vi "AIT 1553 Initialization VI.vi"(8 "error in (no error)":errorcluster, 10 "Custom XML":string, 11 "Device Item Ref in":T1 format="%.0x") -> (0 "error out":errorcluster, 3 "Device Item Ref out":T1 format="%.0x")   [LabVIEW 2011, in "AIT 1553 Custom Device.lvlib"]
uses:
  AIT 1553 Custom Device.lvlib
  <vilib>/NI Veristand/Custom Device API/Custom Device Item Ref.ctl
  Controls and Global/Global.vi
  <vilib>/NI Veristand/Custom Device API/Custom Device API.lvlib
  <vilib>/NI Veristand/Custom Device Tools/Custom Device Utility Library/Custom Device Utility Library.lvlib
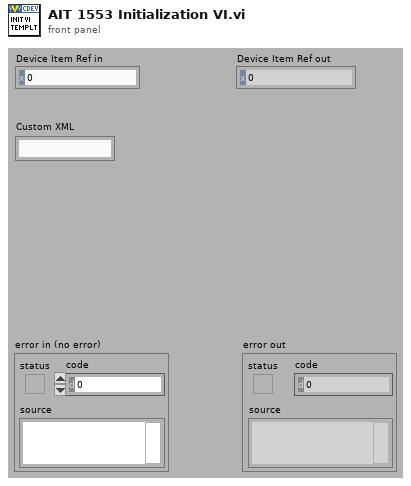
[diagram p1: front panel]
types:
  T1 = typedef "Custom Device API.lvlib/Custom Device Item Ref.ctl" = u64
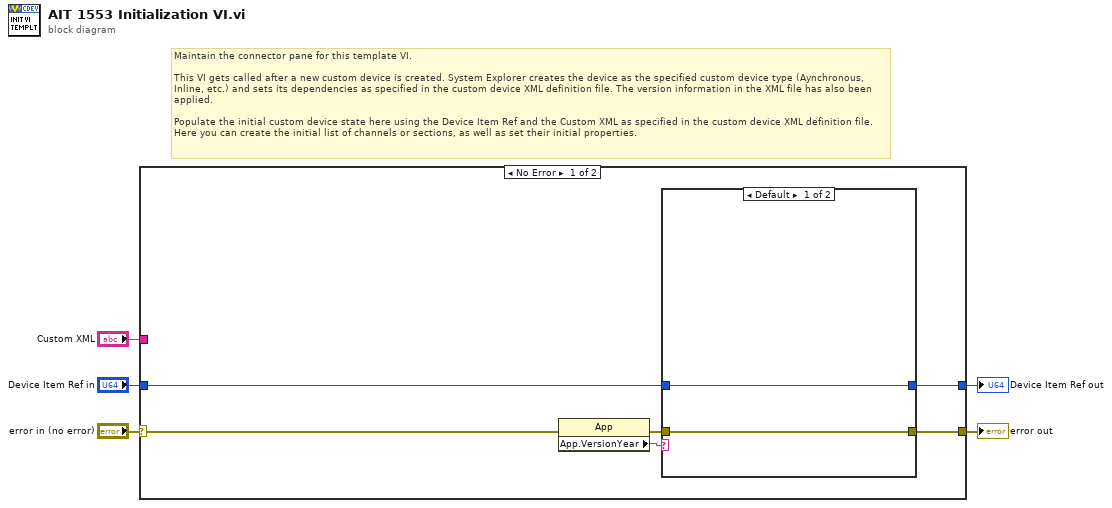
[diagram p0: block diagram]
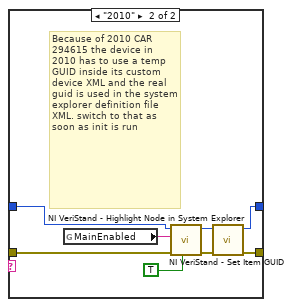
[diagram p2: hidden frame]
diagram:
  # "Maintain the connector pane for this template VI.\n\nThis VI gets called after a new custom device is created. System Explorer creates the device as the specified custom device type (Aynchronous, Inline, etc.) and sets its dependencies as specified in the custom device XML definition file. The version information in the XML file has also been applied.\n\nPopulate the initial custom device state here using the Device Item Ref and the Custom XML as specified in the custom device XML definition file. Here you can create the initial list of channels or sections, as well as set their initial properties."
  n1 = case shown="No Error" "error in (no error)" {
    selector: "error in (no error)" -> [w8 w23]
    tunnel: [w10 w22] -> w4
    tunnel: "Device Item Ref in" -> [w6 w22]
    tunnel: "Custom XML" -> [_ _]
    tunnel: [w11 w23] -> w1
    frame No Error {
      n2 = property class="App"(error in=w8) -> (error out=w7:errorcluster, "App.VersionYear"=w9:string)  [unwired: 1 in, 1 out]
      n3 = case shown="Default" w9 {
        tunnel: w6 -> [w12 w21]
        tunnel: [w12 w17] -> w10
        tunnel: [w13 w14] -> w11
        tunnel: w7 -> [w13 w15]
        frame Default {
        }
        frame "2010" {
          # "Because of 2010 CAR 294615 the device in 2010 has to use a temp GUID inside its custom device XML and the real guid is used in the system explorer definition file XML. switch to that as soon as init is run"
          n4 = global read "Global.vi" "MainEnabled"() -> (w20:string)
          n5 = call <vilib>:"NI VeriStand - Set Item GUID.vi"("Refresh System Explorer Tree? (F)"=TRUE, "error in (no error)"=w15, "GUID"=w20, "Item Ref in"=w21) -> ("error out"=w19:errorcluster, "Item Ref out"=w18:T1)  [unwired: 6 in]
          n6 = call <vilib>:"NI VeriStand - Highlight Node in System Explorer.vi"("error in (no error)"=w19, "Item Ref in"=w18) -> ("error out"=w14:errorcluster, "Node Ptr dup"=w17:T1)  [unwired: 8 in]
        }
      }
    }
    frame Error {
    }
  }
  "error out" <- w1
  "Device Item Ref out" <- w4
